vi "Update Timing.vi"(8 "error in (no error)":errorcluster, 10 "dt(sec)":dbl, 11 "FFT Ref In":refnum<class "FFT.lvclass">) -> (0 "error out":errorcluster, 3 "FFT Ref Out":refnum<class "FFT.lvclass">)   [LabVIEW 2023, in "FFT.lvlib" / "FFT.lvclass"]
uses:
  FFT.lvclass
  C:/Program Files/National Instruments/LabVIEW 2024/vi.lib/FlexLogger/SDK/PluginSDK.lvlibp/PEFClasses/SDK/Processing Element/Processing Element.lvclass
  <vilib>/FlexLogger/SDK/PluginSDK.lvlibp/PEFClasses/SDK/Processing Element/Read System Interface.vi
  <vilib>/FlexLogger/SDK/PluginSDK.lvlibp/PEFClasses/SDK/System Interface/System Interface.lvclass
  <vilib>/FlexLogger/SDK/PluginSDK.lvlibp
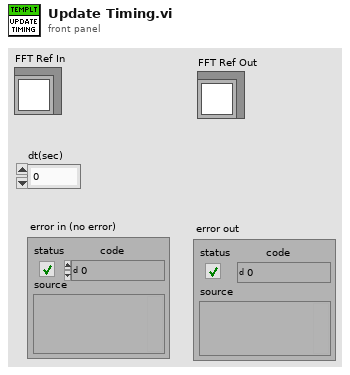
[diagram p1: front panel]
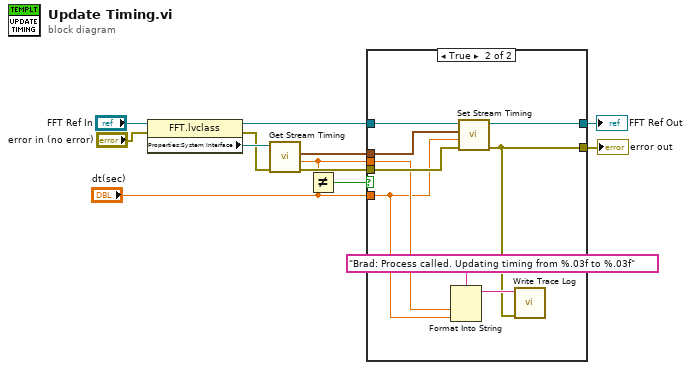
[diagram p0: block diagram]
diagram:
  n1 = property class="FFT.lvclass"(reference="FFT Ref In", error in="error in (no error)") -> (reference out=w7:refnum<class "FFT.lvclass">, error out=w9:errorcluster, "Properties:System Interface"=w11:refnum<class "System Interface.lvclass">)
  n2 = call-dynamic "Get Stream Timing.vi"("error in (no error)"=w9, "System Interface in"=w11) -> ("error out"=w10:errorcluster, "dt(sec)"=w1:dbl, "start time"=w12:timestamp)  [unwired: 6 in, 1 out]
  n3 = Not Equal?(x=w1, y="dt(sec)") -> (x != y?=w6:bool)
  n4 = case shown="True" w6 {
    tunnel: w12 -> [_ w22]
    tunnel: w10 -> [w13 w20]
    tunnel: w7 -> [w14 w23]
    tunnel: "dt(sec)" -> [_ w16]
    tunnel: [w14 w21] -> w4
    tunnel: [w13 w15] -> w2
    tunnel: w1 -> [_ w17]
    frame False {
    }
    frame True {
      n5 = Format Into String(format string="Brad: Process called. Updating timing from %.03f to %.03f" ("Message"), w17, w16) -> (resulting string=w18:string)  [unwired: 2 in, 1 out]
      n6 = call-dynamic "Set Stream Timing.vi"("error in (no error)"=w20, "dt(sec)"=w16, "Start Time"=w22, "Plugin in"=w23) -> ("error out"=w15:errorcluster, "Plugin out"=w21:refnum<class "FFT.lvclass">)  [unwired: 6 in]
      n7 = call <vilib>:"Write Trace Log.vi"("error in (no error)"=w15, "Message"=w18) -> ()  [unwired: 9 in, 1 out]
    }
  }
  "FFT Ref Out" <- w4
  "error out" <- w2
